vi "Hardware-DIDriverConfig.vi"() -> (2 "B Configuration":T1 {"Pump Zener Voltage [V]" min=0 max=240 format="%#_13g"; "DI Zener Voltage [V]" min=0 max=100 format="%#_13g"; "Boost Clamp [V]" min=0 max=220 format="%#_13g"; "Boost Voltage [V]" min=0 max=220 format="%#_13g"}, 3 "A Configuration":T1 {"Pump Zener Voltage [V]" min=0 max=240 format="%#_13g"; "DI Zener Voltage [V]" min=0 max=100 format="%#_13g"; "Boost Clamp [V]" min=0 max=220 format="%#_13g"; "Boost Voltage [V]" min=0 max=220 format="%#_13g"})   [LabVIEW 2016, in "DSI-RT.lvlib"]
uses:
  DSI-RT.lvlib
  <vilib>/Powertrain Controls/Device Drivers/DCM/Rev0/FPGA/DI - Bank Configuration.ctl
  <vilib>/Powertrain Controls/Device Drivers/DCM/Rev0/FPGA/DCM - FPGA.lvlib
  <vilib>/Powertrain Controls/Device Drivers/DCM/Rev0/RT/Configuration.ctl
  <vilib>/Powertrain Controls/Device Drivers/DCM/Rev0/RT/DCM - RT.lvclass
panel:
  # "Voltage [DV]"
  # "Voltage [V]"
  # "Voltage [DV]"
  # "Voltage [V]"
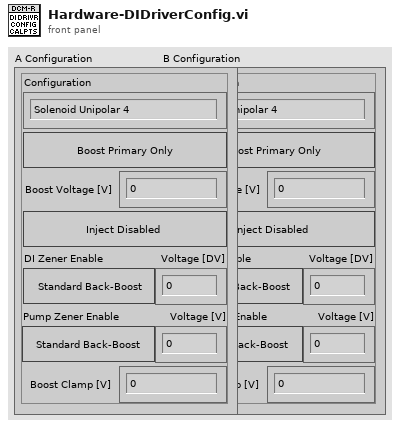
[diagram p1: front panel]
types:
  T1 = typedef "DCM - RT.lvclass/Configuration.ctl" = cluster{"Configuration":T2, "Power Supply Enable":bool, "Boost Voltage [V]":sgl, "Inject Enable":bool, "DI Zener Enable":bool, "DI Zener Voltage [V]":sgl, "Pump Zener Enable":bool, "Pump Zener Voltage [V]":sgl, "Boost Clamp [V]":sgl}
  T2 = typedef "DCM - FPGA.lvlib/DI - Bank Configuration.ctl" = enum8{"Solenoid Unipolar 4", "Solenoid Unipolar 7 (Muxed)", "Solenoid Unipolar 8 (Muxed)", "Solenoid Bipolar 2", "Solenoid Bipolar 3 (Muxed)", "Piezo Unipolar 2", "Piezo Unipolar 3 (Muxed)", "Piezo Unipolar 4 (Muxed)", "Piezo Bipolar 2", "Piezo Bipolar 3 (Muxed)"}
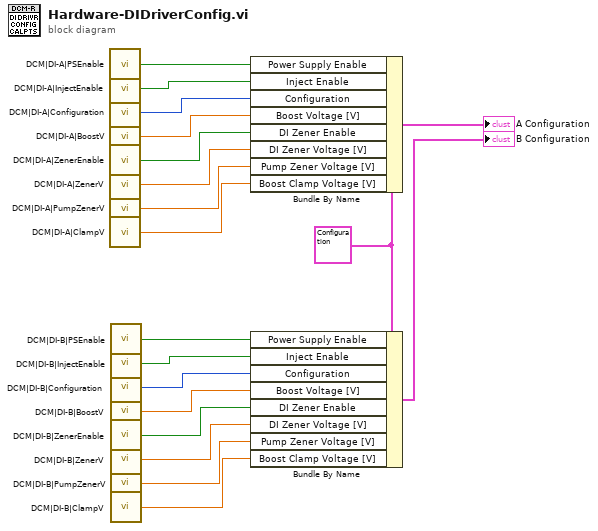
[diagram p0: block diagram]
diagram:
  w17 = T1 {"Configuration"=enum."Solenoid Unipolar 4", "Power Supply Enable"=FALSE, "Boost Voltage [V]"=0.0, "Inject Enable"=FALSE, "DI Zener Enable"=FALSE, "DI Zener Voltage [V]"=0.0, "Pump Zener Enable"=FALSE, "Pump Zener Voltage [V]"=0.0, "Boost Clamp [V]"=0.0} ("A Configuration")
  n1 = call "DCM|DI-A|PSEnable"() -> ("Value"=w1:bool)
  n2 = call "DCM|DI-A|InjectEnable"() -> ("Value"=w2:bool)
  n3 = call "DCM|DI-A|Configuration"() -> ("Value"=w3:u8)
  n4 = call "DCM|DI-A|BoostV"() -> ("Value"=w4:sgl)
  n5 = call "DCM|DI-A|ZenerEnable"() -> ("Value"=w5:bool)
  n6 = call "DCM|DI-A|ZenerV"() -> ("Value"=w6:sgl)
  n7 = call "DCM|DI-A|PumpZenerV"() -> ("Value"=w7:sgl)
  n8 = call "DCM|DI-A|ClampV"() -> ("Value"=w8:sgl)
  n9 = call "DCM|DI-B|PSEnable"() -> ("Value"=w9:bool)
  n10 = call "DCM|DI-B|InjectEnable"() -> ("Value"=w10:bool)
  n11 = call "DCM|DI-B|Configuration"() -> ("Value"=w11:u8)
  n12 = call "DCM|DI-B|BoostV"() -> ("Value"=w12:sgl)
  n13 = call "DCM|DI-B|ZenerEnable"() -> ("Value"=w13:bool)
  n14 = call "DCM|DI-B|ZenerV"() -> ("Value"=w14:sgl)
  n15 = call "DCM|DI-B|PumpZenerV"() -> ("Value"=w15:sgl)
  n16 = call "DCM|DI-B|ClampV"() -> ("Value"=w16:sgl)
  n17 = Bundle By Name(cluster=w17, "Power Supply Enable"=w1, "Inject Enable"=w2, "Configuration"=w3, "Boost Voltage [V]"=w4, "DI Zener Enable"=w5, "DI Zener Voltage [V]"=w6, "Pump Zener Voltage [V]"=w7, "Boost Clamp Voltage [V]"=w8) -> (→"A Configuration":T1)
  n18 = Bundle By Name(cluster=w17, "Power Supply Enable"=w9, "Inject Enable"=w10, "Configuration"=w11, "Boost Voltage [V]"=w12, "DI Zener Enable"=w13, "DI Zener Voltage [V]"=w14, "Pump Zener Voltage [V]"=w15, "Boost Clamp Voltage [V]"=w16) -> (→"B Configuration":T1)
